vi "Constructor.vi"(8 "error in (no error)":errorcluster, 11 "Keithley 2400 in":refnum<class "Keithley 2400.lvclass">) -> (0 "error out":errorcluster, 2 "Init":bool, 3 "Keithley 2400 out":refnum<class "Keithley 2400.lvclass">)   [LabVIEW 2011, in "Keithley 2400.lvclass"]
uses:
  Keithley 2400.lvclass
  Keithley 2400.lvclass/Keithley 2400.ctl
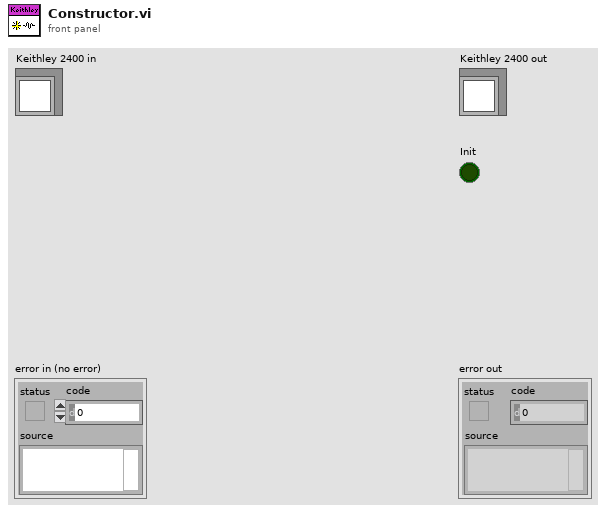
[diagram p1: front panel]
types:
  T1 = cluster{"status":bool, "code":bool, "source":bool}
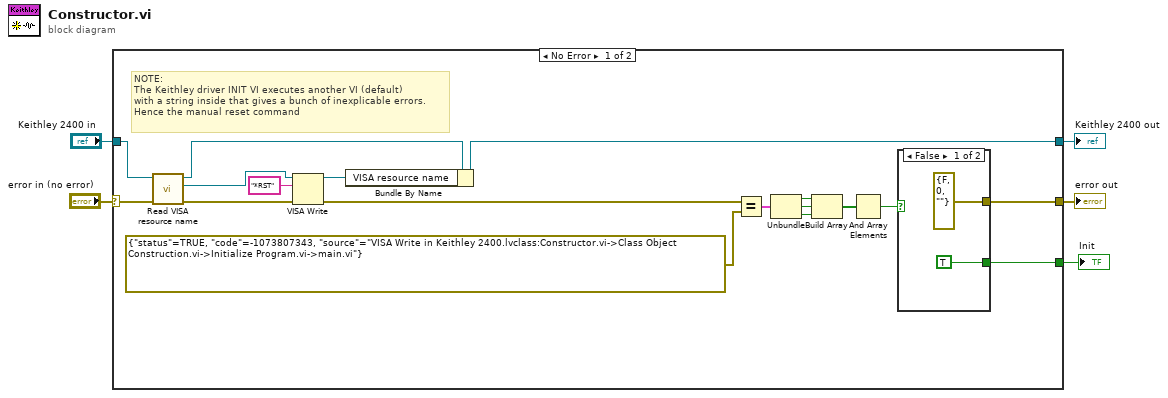
[diagram p0: block diagram]
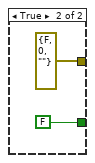
[diagram p2: hidden frame]
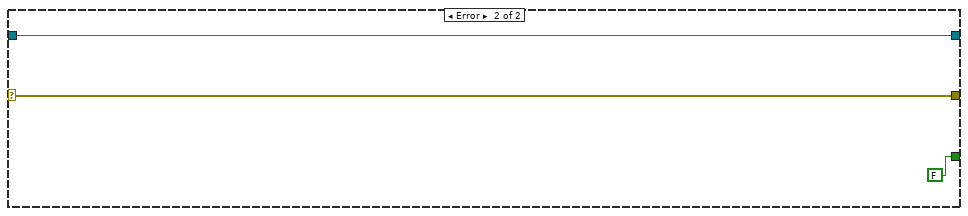
[diagram p3: hidden frame]
diagram:
  n1 = case shown="No Error" "error in (no error)" {
    selector: "error in (no error)" -> [w19 w30]
    tunnel: [w7 w30] -> w4
    tunnel: [w23 w29] -> w2
    tunnel: "Keithley 2400 in" -> [w20 w29]
    tunnel: [w6 FALSE] -> w1
    frame No Error {
      # "NOTE:\nThe Keithley driver INIT VI executes another VI (default)\nwith a string inside that gives a bunch of inexplicable errors.\nHence the manual reset command"
      n2 = call-dynamic "Read VISA resource name.vi"("error in (no error)"=w19, "Power Supply in"=w20) -> ("error out"=w18:errorcluster, "VISA resource name"=w16:refnum<visa-resource-name>, "Power Supply out"=w17:refnum<class "Keithley 2400.lvclass">)  [unwired: 7 in]
      n3 = VISA Write(VISA resource name=w16, write buffer="*RST" ("Reset Command"), error in (no error)=w18) -> (VISA resource name out=w21:refnum<visa-resource-name>, error out=w15:errorcluster)  [unwired: 1 out]
      n4 = Bundle By Name(cluster=w17, "VISA resource name"=w21) -> (w23:refnum<class "Keithley 2400.lvclass">)
      n5 = Equal?(x=w15, y=errorcluster {"status"=TRUE, "code"=-1073807343, "source"="VISA Write in Keithley 2400.lvclass:Constructor.vi->Class Object Construction.vi->Initialize Program.vi->main.vi"} ("error out 2")) -> (x = y?=w13:T1)
      n6 = Unbundle(w13) -> ("status"=w12:bool, "code"=w11:bool, "source"=w10:bool)
      n7 = Build Array(w12, w11, w10) -> (w9:bool[])
      n8 = And Array Elements(Boolean array=w9) -> (logical AND=w8:bool)
      n9 = case shown="False" w8 {
        tunnel: [errorcluster {"status"=FALSE, "code"=0, "source"=""} ("error in (no error) 2") errorcluster {"status"=FALSE, "code"=0, "source"=""} ("error in (no error) 2")] -> w7
        tunnel: [TRUE FALSE] -> w6
        frame False {
        }
        frame True {
        }
      }
    }
    frame Error {
    }
  }
  "error out" <- w4
  "Keithley 2400 out" <- w2
  "Init" <- w1
